vi "scorecaddy_datalogger.vi"() -> ()   [LabVIEW 2018]
uses:
  control/enumBaseFunction.ctl
  <vilib>/Instr/_visa.llb/VISA Configure Serial Port (Instr).vi
panel:
  out "라벨":string
  in  "5":bool
  in  "4":bool
  in  "3":bool
  out "라벨값":i32
  in  "2":bool
  in  "1":bool
  in  "0":bool
  out "데이터용량(byte)":i64
  out "데이터개수":i32
  in  "파일명":string
  in  "파일저장":bool
  out "tick(20ms)":dbl[](graph)
  out "acc":dbl[][](graph)
  out "gyro":dbl[][](graph)
  out "큐처리시간":u32(graph)
  out "버퍼된 바이트수":u32(graph)
  out "수신바이트":i32(graph)
  out "BLE수신시간":u32(graph)
  out "버퍼 읽기":string
  in  "정지":bool
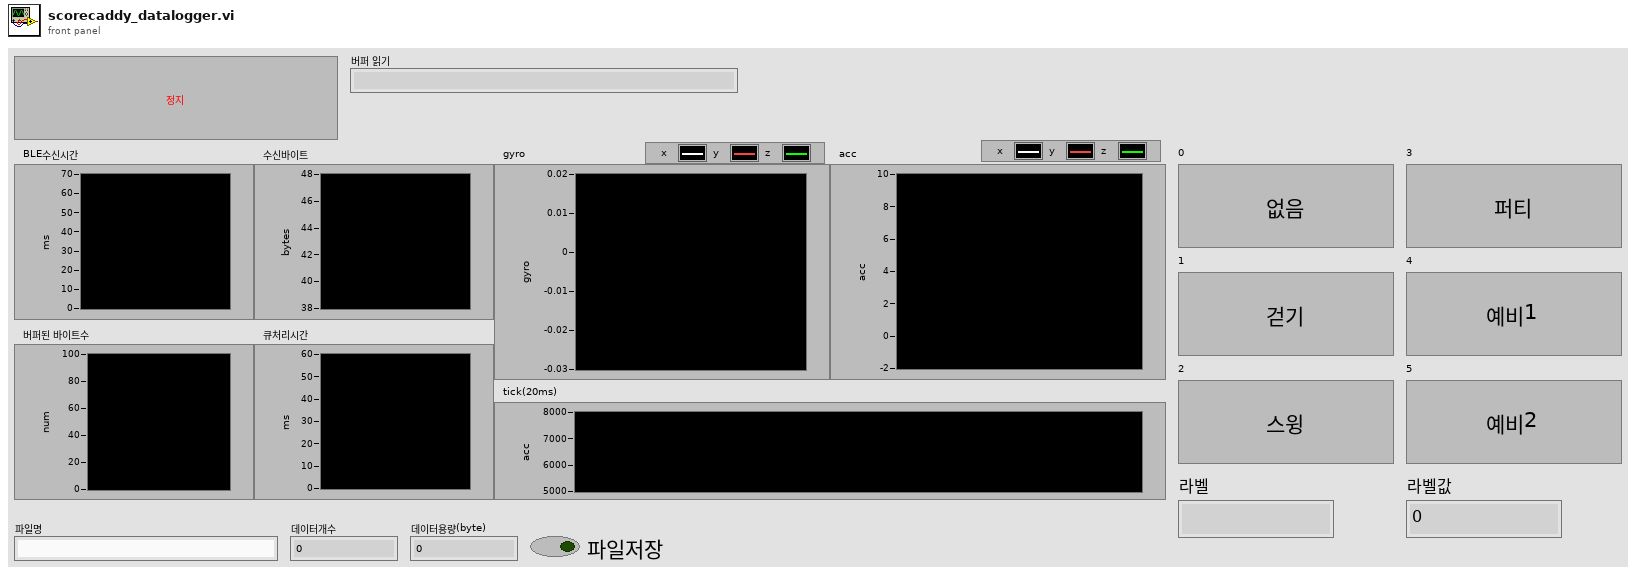
[diagram p1: front panel]
types:
  T1 = typedef "enumBaseFunction.ctl" = enum16{"열기", "쓰기", "확인", "닫기"}
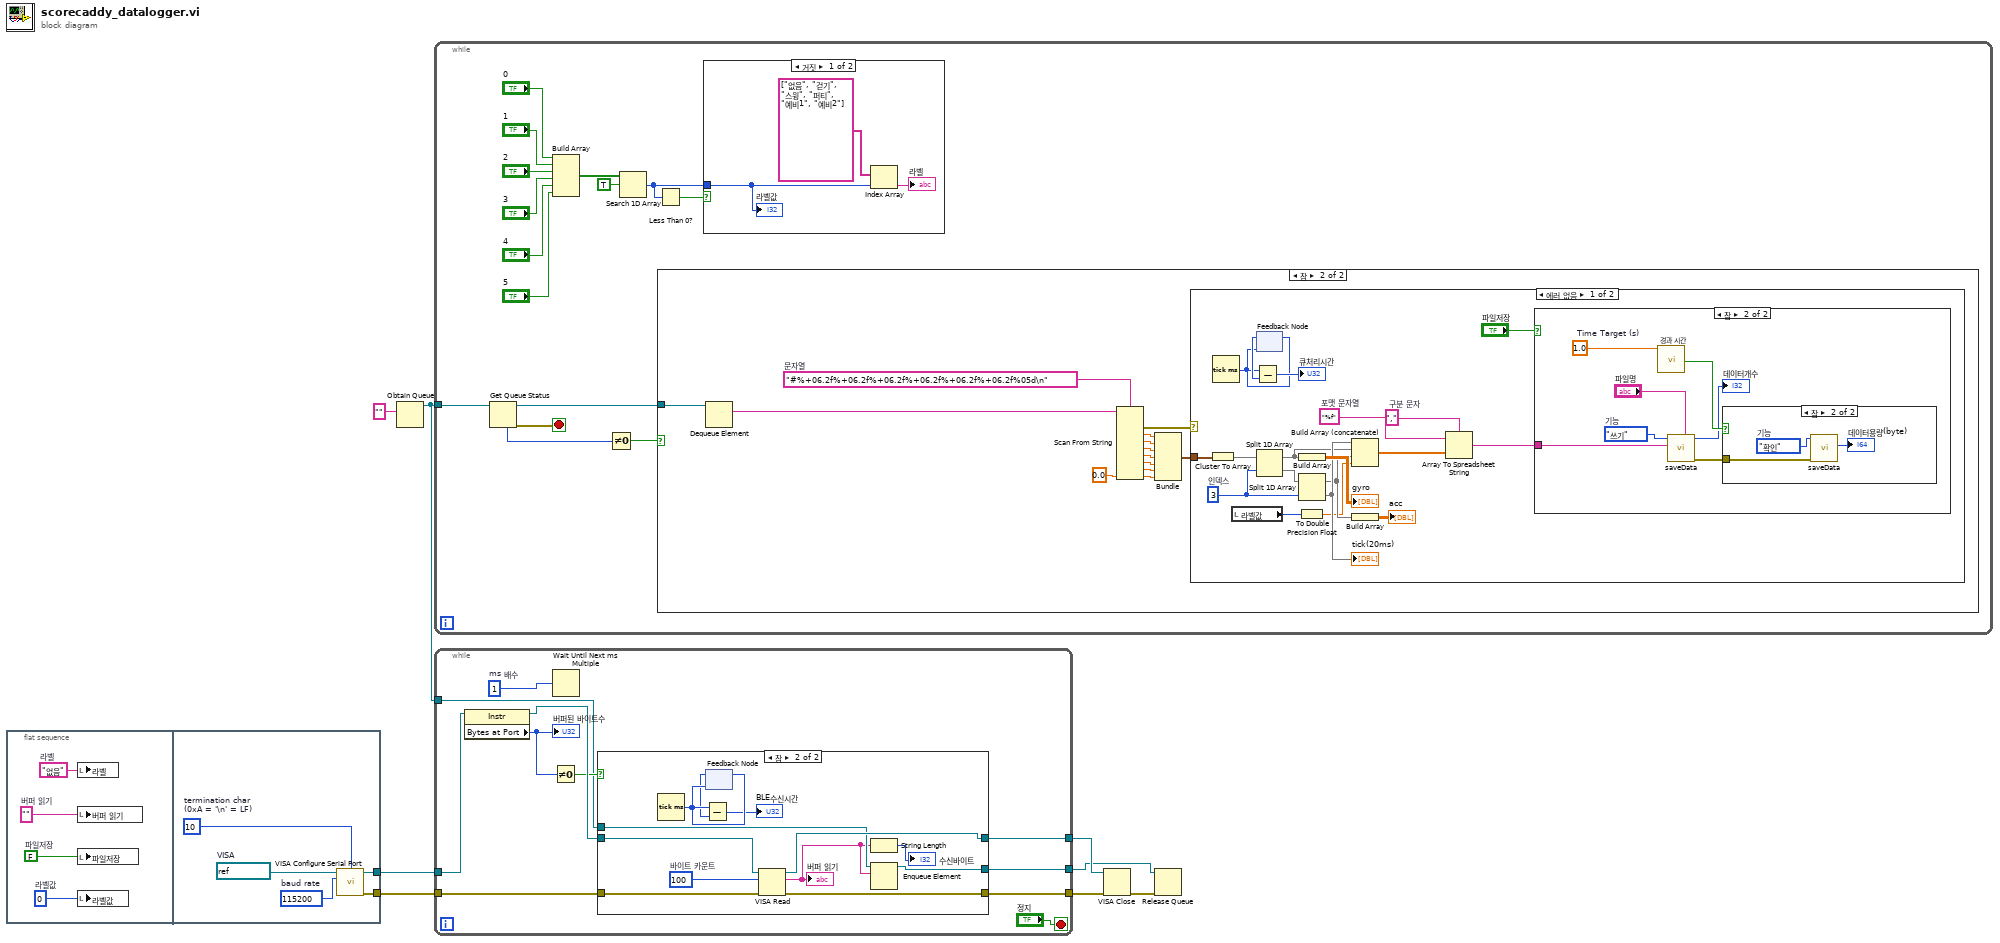
[diagram p0: block diagram]
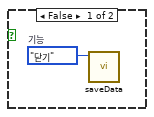
[diagram p4: hidden frame]
diagram:
  n1 = flat-sequence {
    tunnel: [w17] -> w8
    tunnel: [w16] -> w7
    frame #0 {
      w9 = 0  # 라벨값
      w10 = "없음"  # 라벨
      w11 = FALSE  # 파일저장
      w12 = ""  # 버퍼 읽기
      n2 = local write "라벨"(w10) -> ()
      n3 = local write "버퍼 읽기"(w12) -> ()
      n4 = local write "파일저장"(w11) -> ()
      n5 = local write "라벨값"(w9) -> ()
    }
    frame #1 {
      w14 = u8 10  # termination char (0xA = '\n' = LF)
      w13 = u32 115200  # baud rate
      w15 = refnum<visa-resource-name> "COM9"  # VISA
      n6 = call-poly "VISA Configure Serial Port"("VISA resource name"=w15, "termination char\n(0xA = '\\n' = LF)"=w14, "baud rate (9600)"=w13) -> ("VISA resource name out"=w17:refnum<visa-resource-name>, "error out"=w16:errorcluster)  [unwired: 11 in]
    }
  }
  n7 = Obtain Queue(element data type="") -> (queue out=w4:refnum<queue>)  [unwired: 4 in, 2 out]
  n8 = while {
    tunnel: w4 -> [w32]
    stop <- w28 stop-if-true
    n9 = Get Queue Status(queue=w32) -> (queue out=w29:refnum<queue>, error out=w28:errorcluster, # elements in queue=w31:i32)  [unwired: 2 in, 5 out]
    n10 = Build Array("0", "1", "2", "3", "4", "5") -> (w21:bool[])
    n11 = Not Equal To 0?(x=w31) -> (x != 0?=w30:bool)
    n12 = Search 1D Array(1D array=w21, element=TRUE) -> (index of element=w19:i32)  [unwired: 1 in]
    n13 = Less Than 0?(x=w19) -> (x < 0?=w18:bool)
    n14 = case shown="참" w30 {
      tunnel: w29 -> [_ w48]
      frame False {
      }
      frame True {
        w46 = "#%+06.2f%+06.2f%+06.2f%+06.2f%+06.2f%+06.2f%05d\n"  # 문자열
        n15 = Dequeue Element(queue=w48) -> (element=w47:string)  [unwired: 2 in, 3 out]
        n16 = Scan From String(format string=w46, input string=w47, default 7=0.0) -> (error out=w45:errorcluster, output 1=w44:dbl, output 2=w43:dbl, output 3=w42:dbl, output 4=w41:dbl, output 5=w40:dbl, output 6=w39:dbl, output 7=w38:dbl)  [unwired: 8 in, 2 out]
        n17 = Bundle(w44, w43, w42, w41, w40, w39, w38) -> (w37:cluster{dbl, dbl, dbl, dbl, dbl, dbl, dbl})  [unwired: 1 in]
        n18 = case shown="에러 없음" w45 {
          tunnel: w37 -> [w64 _]
          frame No Error {
            w53 = "%f"  # 포맷 문자열
            w54 = ","  # 구분 문자
            w61 = 3  # 인덱스
            n19 = Cluster To Array(cluster=w64) -> (array=w63:dbl[])
            n20 = Tick Count (ms)() -> (millisecond timer value=w65:u32)
            n21 = local read "라벨값"() -> (w50:i32)
            n22 = feedback #1(w65) -> (w66:u32)
            n23 = Subtract(x=w65, y=w66) -> (x-y=→"큐처리시간":u32)
            n24 = feedback-in #1(w65) -> ()
            n25 = Split 1D Array(array=w63, index=w61) -> (first subarray=w57:dbl[], second subarray=w62:dbl[])
            n26 = Build Array(w57) -> (→"gyro":dbl[][])
            n27 = Split 1D Array(array=w62, index=w61) -> (first subarray=w56:dbl[], second subarray=w58:dbl[])
            "tick(20ms)" <- w58
            n28 = To Double Precision Float(number=w50) -> (double precision float=w49:dbl)
            n29 = Build Array (concatenate)(w58, w57, w56, w49) -> (w55:dbl[])
            n30 = Build Array(w56) -> (→"acc":dbl[][])
            n31 = Array To Spreadsheet String(delimiter (Tab)=w54, array=w55, 3:w53) -> (spreadsheet string=w52:string)
            n32 = case shown="참" "파일저장" {
              tunnel: w52 -> [_ w71]
              frame False {
                w68 = enumBaseFunction."닫기"  # 기능
                n33 = call "saveData.vi"("기능"=w68) -> ()  [unwired: 8 in, 3 out]
              }
              frame True {
                w73 = enumBaseFunction."쓰기"  # 기능
                w75 = 1.0  # Time Target (s)
                n34 = call "경과 시간"("Time Target (s)"=w75) -> ("Time has Elapsed"=w74:bool)  [unwired: 11 in, 7 out]
                n35 = call "saveData.vi"("파일명"="파일명", "데이터"=w71, "기능"=w73) -> ("error out"=w72:errorcluster, "데이터개수"=→"데이터개수":i32)  [unwired: 6 in, 1 out]
                n36 = case shown="참" w74 {
                  tunnel: w72 -> [_ w78]
                  frame False {
                  }
                  frame True {
                    w77 = enumBaseFunction."확인"  # 기능
                    n37 = call "saveData.vi"("error in"=w78, "기능"=w77) -> ("데이터용량(byte)"=→"데이터용량(byte)":i64)  [unwired: 7 in, 2 out]
                  }
                }
              }
            }
          }
          frame Error {
          }
        }
      }
    }
    n38 = case shown="거짓" w18 {
      tunnel: w19 -> [w33 _]
      frame False {
        n39 = Index Array(array=string[] ["없음", "걷기", "스윙", "퍼티", "예비1", "예비2"], index=w33) -> (element=→"라벨":string)
        "라벨값" <- w33
      }
      frame True {
      }
    }
  }
  n40 = while {
    tunnel: w8 -> [w88]
    tunnel: w7 -> [w87]
    tunnel: [w86] -> w6
    tunnel: [w85] -> w5
    tunnel: w4 -> [w80]
    tunnel: [w79] -> w2
    stop <- "정지" stop-if-true
    w81 = u32 1  # ms 배수
    n41 = property class="Instr"(reference=w88) -> (reference out=w84:refnum<visa-resource-name>, "Bytes at Port"=w82:u32)  [unwired: 1 in, 1 out]
    "버퍼된 바이트수" <- w82
    n42 = Not Equal To 0?(x=w82) -> (x != 0?=w83:bool)
    n43 = Wait Until Next ms Multiple(millisecond multiple=w81) -> ()  [unwired: 1 out]
    n44 = case shown="참" w83 {
      tunnel: w87 -> [w92 w104]
      tunnel: [w91 w103] -> w86
      tunnel: [w92 w102] -> w85
      tunnel: w84 -> [w91 w101]
      tunnel: [w90 w93] -> w79
      tunnel: w80 -> [w90 w95]
      frame False {
      }
      frame True {
        w100 = u32 100  # 바이트 카운트
        n45 = Tick Count (ms)() -> (millisecond timer value=w99:u32)
        n46 = feedback #2(w99) -> (w98:u32)
        n47 = Subtract(x=w99, y=w98) -> (x-y=→"BLE수신시간":u32)
        n48 = feedback-in #2(w99) -> ()
        n49 = VISA Read(VISA resource name=w101, byte count=w100, error in (no error)=w104) -> (VISA resource name out=w103:refnum<visa-resource-name>, read buffer=w94:string, error out=w102:errorcluster)  [unwired: 1 out]
        "버퍼 읽기" <- w94
        n50 = String Length(string=w94) -> (length=→"수신바이트":i32)
        n51 = Enqueue Element(queue=w95, element=w94) -> (queue out=w93:refnum<queue>)  [unwired: 2 in, 2 out]
      }
    }
  }
  n52 = VISA Close(VISA resource name=w6, error in (no error)=w5) -> (error out=w3:errorcluster)
  n53 = Release Queue(queue=w2, error in (no error)=w3) -> ()  [unwired: 1 in, 3 out]
